vi "Close Notifiers.vi"(8 "error in (no error)":errorcluster, 11 "Notifiers":T1) -> (0 "error out":errorcluster)   [LabVIEW 2015]
uses:
  Notifier.ctl
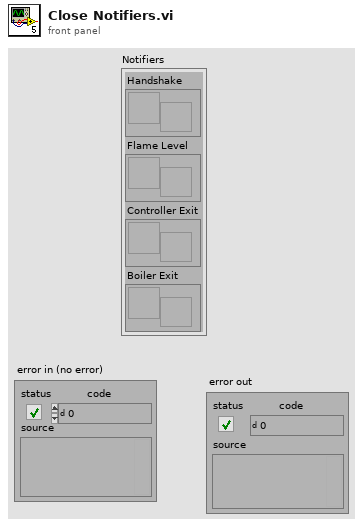
[diagram p1: front panel]
types:
  T1 = typedef "Notifier.ctl" = cluster{"Handshake":refnum<notifier>, "Flame Level":refnum<notifier>, "Controller Exit":refnum<notifier>, "Boiler Exit":refnum<notifier>}
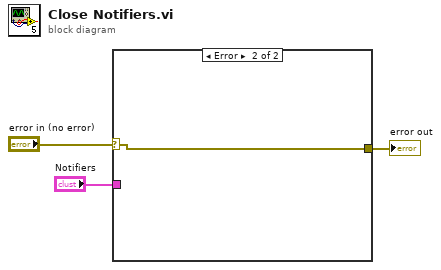
[diagram p0: block diagram]
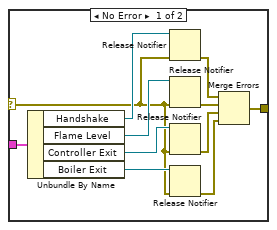
[diagram p2: hidden frame]
diagram:
  n1 = case shown="Error" "error in (no error)" {
    selector: "error in (no error)" -> [w9 w15]
    tunnel: "Notifiers" -> [w14 _]
    tunnel: [w4 w15] -> w1
    frame No Error {
      n2 = Unbundle By Name(w14) -> ("Handshake"=w13:refnum<notifier>, "Flame Level"=w12:refnum<notifier>, "Controller Exit"=w11:refnum<notifier>, "Boiler Exit"=w10:refnum<notifier>)
      n3 = Release Notifier(notifier=w13, error in (no error)=w9) -> (error out=w8:errorcluster)  [unwired: 1 in, 2 out]
      n4 = Release Notifier(notifier=w12, error in (no error)=w9) -> (error out=w7:errorcluster)  [unwired: 1 in, 2 out]
      n5 = Release Notifier(notifier=w11, error in (no error)=w9) -> (error out=w6:errorcluster)  [unwired: 1 in, 2 out]
      n6 = Release Notifier(notifier=w10, error in (no error)=w9) -> (error out=w5:errorcluster)  [unwired: 1 in, 2 out]
      n7 = Merge Errors(w8, w7, w6, w5) -> (w4:errorcluster)
    }
    frame Error {
    }
  }
  "error out" <- w1
